vi "loadActionPanelFromPath.vi"(8 "error in (no error)":errorcluster, 10 "ActionPanel in":refnum<class "ActionPanel.lvclass">, 11 "ActionEditor in":refnum<class "ActionEditor.lvclass">) -> (0 "error out":errorcluster, 3 "ActionEditor out":refnum<class "ActionEditor.lvclass">)   [LabVIEW 2009, in "Views.lvlib" / "ScriptEditor.lvlib" / "ActionEditor.lvclass"]
uses:
  ActionEditor.lvclass
  ActionPanels/ActionPanel.lvclass
  ActionEditor.lvclass/ActionEditor.ctl
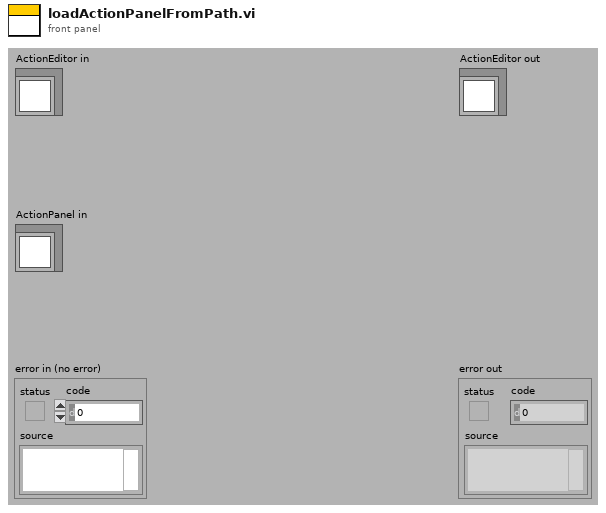
[diagram p1: front panel]
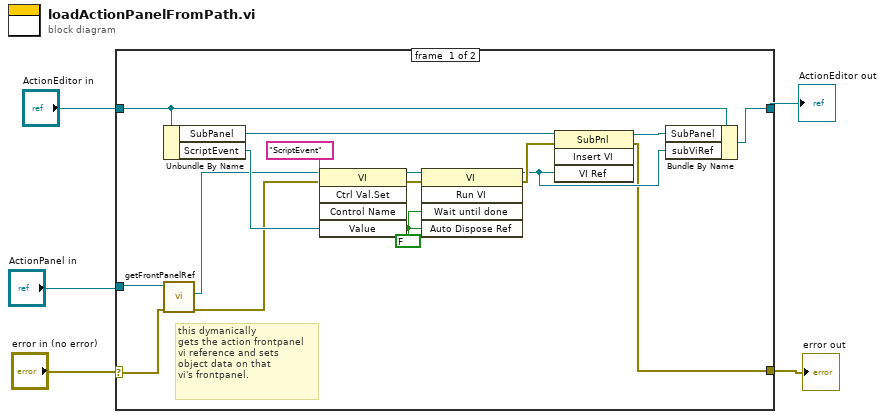
[diagram p0: block diagram]
diagram:
  n1 = case shown="No Error" "error in (no error)" {
    selector: "error in (no error)" -> [w8 w23]
    tunnel: [w11 w23] -> w4
    tunnel: [w12 w22] -> w2
    tunnel: "ActionEditor in" -> [w19 w22]
    tunnel: "ActionPanel in" -> [w9 _]
    frame #0 {
      w14 = FALSE
      # "this dymanically\ngets the action frontpanel \nvi reference and sets\nobject data on that\nvi's frontpanel."
      n2 = Unbundle By Name(w19) -> ("SubPanel"=w18:refnum<vi>, "ScriptEvent"=w10:refnum<class "ScriptEvent.lvclass">)
      n3 = call-dynamic "getFrontPanelRef.vi"("error in (no error)"=w8, "ActionPanel in"=w9) -> ("error out"=w6:errorcluster, "vi reference"=w7:refnum<vi>)  [unwired: 7 in, 1 out]
      n4 = invoke class="VI" method="Ctrl Val.Set"(reference=w7, error in=w6, "Control Name"="ScriptEvent", "Value"=w10) -> (reference out=w17:refnum<vi>, error out=w16:errorcluster)  [unwired: 1 in, 3 out]
      n5 = invoke class="VI" method="Run VI"(reference=w17, error in=w16, "Wait until done"=w14, "Auto Dispose Ref"=w14) -> (reference out=w13:refnum<vi>, error out=w15:errorcluster)  [unwired: 1 in, 3 out]
      n6 = invoke class="SubPnl" method="Insert VI"(reference=w18, error in=w15, "VI Ref"=w13) -> (reference out=w20:refnum<vi>, error out=w11:errorcluster)  [unwired: 1 in, 2 out]
      n7 = Bundle By Name(cluster=w19, "SubPanel"=w20, "subViRef"=w13) -> (w12:refnum<class "ActionEditor.lvclass">)
    }
    frame #1 {
    }
  }
  "error out" <- w4
  "ActionEditor out" <- w2
